vi "Calibrate ECU Torque DutyCycle.vi"(7 "CaliTorque_Bypass Calibration":bool, 11 "ECU Torque DutyCycle":dbl) -> (3 "Calibrated ECU Torque DutyCycle":dbl)   [LabVIEW 2018]
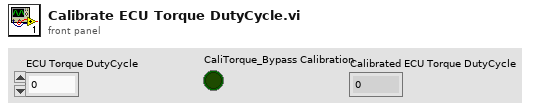
[diagram p1: front panel]
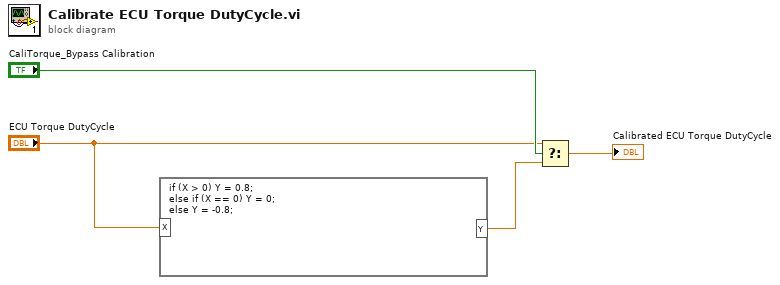
[diagram p0: block diagram]
diagram:
  n1 = formula code="if (X > 0) Y = 0.8;\nelse if (X == 0) Y = 0;\nelse Y = -0.8;"("X"="ECU Torque DutyCycle") -> ("Y"=w4:dbl)
  n2 = Select(t="ECU Torque DutyCycle", s="CaliTorque_Bypass Calibration", f=w4) -> (s? t:f=→"Calibrated ECU Torque DutyCycle":dbl)
